vi "Configure Channel Binding.vi"(8 "error in (no error)":errorcluster, 9 "NIVS.System Definition Root":refnum<k24>, 11 "Data cluster in":T1) -> (0 "error out":errorcluster, 3 "Data cluster out":T1)   [LabVIEW 2013]
doc: "Use this template to create a dialog box with event handling."
uses:
  <vilib>/NI Veristand/UI Controls/Single Node Browser/NI_VS UI Single Node Browser.lvlib
  NationalInstruments.VeriStand.SystemStorage
  Support/PWM Object Parameters.ctl
  NationalInstruments.VeriStand.SystemStorageUI
panel:
  in  "RIO?":bool caption="Hardware type - click to toggle"
  in  "Cancel":bool
  in  "Ok":bool
  in  "Selected Channel":refnum<k24>(container)
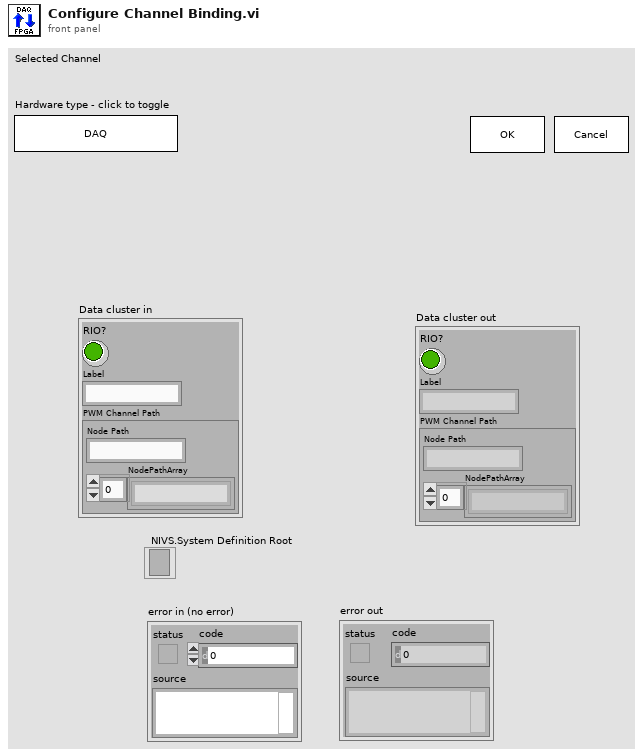
[diagram p1: front panel]
types:
  T1 = typedef "PWM Object Parameters.ctl" = cluster{"RIO?":bool, "Label":string, "PWM Channel Path":cluster{"NodePathArray":string[], "Node Path":string}}
  T2 = typedef "NI_VS UI Single Node Browser.lvlib/Callback Type.ctl" = cluster{"Net Callbacks":refnum<k27>[], "Event":refnum<user-event>}
  T3 = typedef "NI_VS UI Single Node Browser.lvlib/Node Ref.ctl" = refnum<k24>
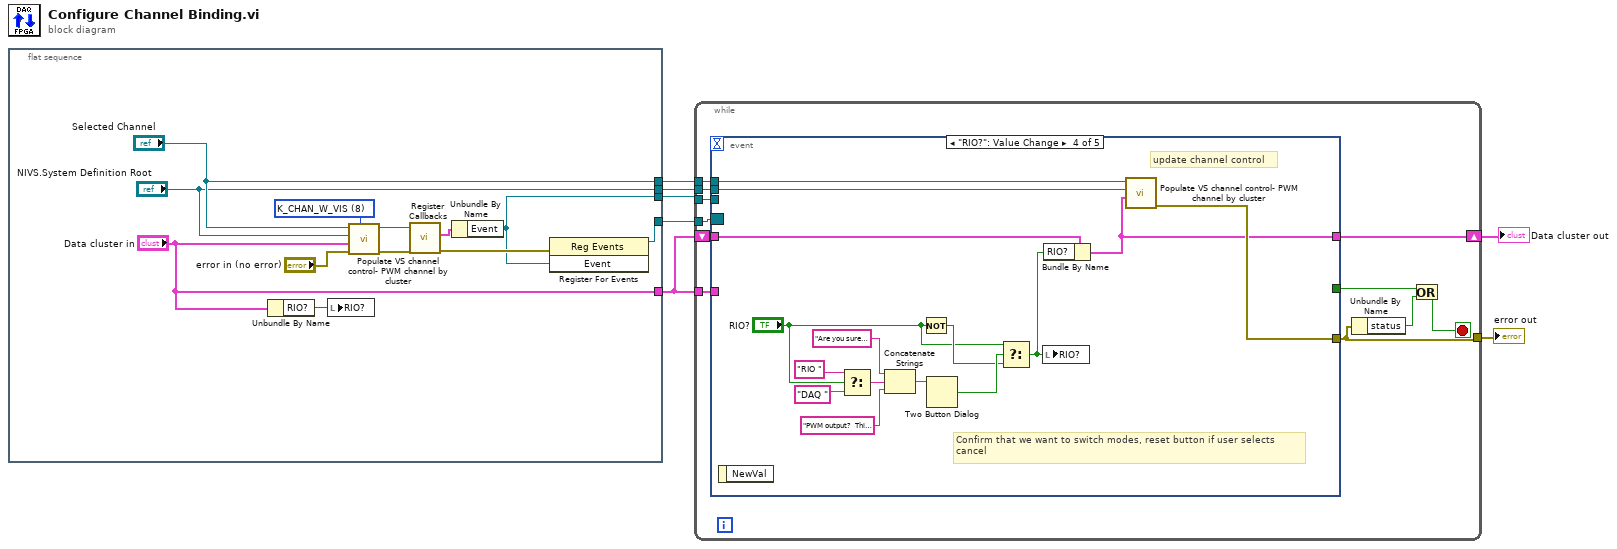
[diagram p0: block diagram]
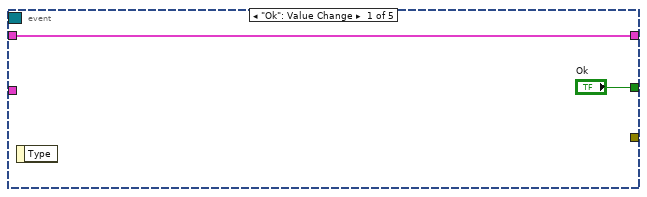
[diagram p2: hidden frame]
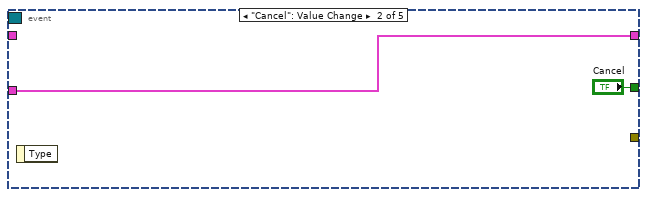
[diagram p3: hidden frame]
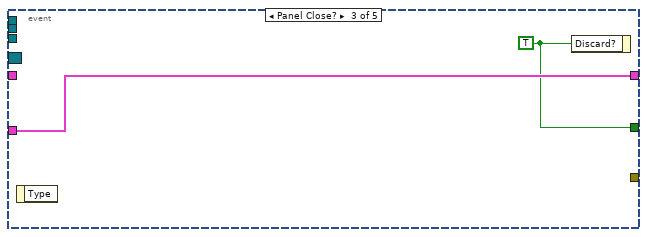
[diagram p4: hidden frame]
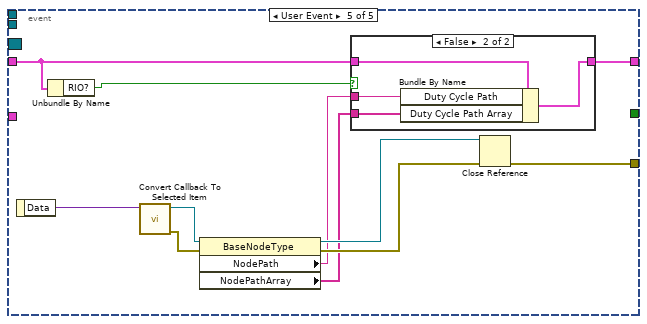
[diagram p5: hidden frame]
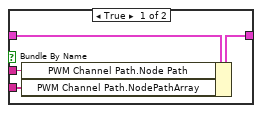
[diagram p6: hidden frame]
diagram:
  n1 = flat-sequence {
    tunnel: [w18] -> w6
    tunnel: [w13] -> w4
    tunnel: ["Selected Channel"] -> w3
    tunnel: ["NIVS.System Definition Root"] -> w2
    tunnel: ["Data cluster in"] -> w1
    frame #0 {
      w10 = u8 8 items=["K_CHAN_R", "K_CHAN_W", "K_CHAN_RW", "K_CHAN_VOLT", "K_CHAN_FAULT", "K_ALL", "K_CUSTOM", "K_CHAN_R_VIS", "K_CHAN_W_VIS", "K_CHAN_RW_VIS", "K_CHAN_VOLT_VIS", "K_CHAN_FAULT_VIS"] ("DisplayFilter")
      n2 = Unbundle By Name("Data cluster in") -> ("RIO?"=w8:bool)
      n3 = local write "RIO?"(w8) -> ()
      n4 = call "Populate VS channel control- PWM channel by cluster.vi"("DisplayFilter"=w10, "error in (no error)"="error in (no error)", "Data cluster in"="Data cluster in", "NIVS.System Definition Root"="NIVS.System Definition Root", ".NET Refnum in"="Selected Channel") -> ("error out"=w15:errorcluster, ".NET Refnum out"=w14:refnum<k24>)  [unwired: 5 in]
      n5 = call <vilib>:"Register Callbacks.vi"("error in (no error)"=w15, "Single Node Browser"=w14) -> ("error out"=w19:errorcluster, "Callbacks"=w16:T2)  [unwired: 7 in, 1 out]
      n6 = Unbundle By Name(w16) -> ("Event"=w13:refnum<user-event>)
      n7 = register-events(error in=w19, w13) -> (reference out=w18:refnum<event-registration>)  [unwired: 1 in, 1 out]
    }
  }
  n8 = while {
    tunnel: [w29] -> w7
    tunnel: w6 -> [w27]
    shift-right: [w24] -> w5
    shift-left: w1 -> [w26]
    tunnel: w1 -> [w25]
    tunnel: w4 -> [w22]
    tunnel: w3 -> [w21]
    tunnel: w2 -> [w20]
    stop <- w23 stop-if-true
    n9 = event shown="[3] \"RIO?\": Value Change" {
      selector: w27 -> [_ _ _ _ _]
      dyn-events: _ -> [_ _ _ _ _]
      timeout: _ -> [_ _ _ _ _]
      tunnel: ["Ok" "Cancel" w35 _ _] -> w30
      tunnel: [_ _ _ w44 w61] -> w29
      tunnel: w26 -> [w31 _ _ w45 w53]
      tunnel: w25 -> [_ w33 w36 _ _]
      tunnel: [w31 w33 w36 w43 w56] -> w24
      tunnel: w22 -> [_ _ _ _ _]
      tunnel: w21 -> [_ _ _ w47 _]
      tunnel: w20 -> [_ _ _ w46 _]
      event "Ok": Value Change {
        n10 = event-data() -> ()  [unwired: 1 in, 1 out]
      }
      event "Cancel": Value Change {
        n11 = event-data() -> ()  [unwired: 1 in, 1 out]
      }
      event Panel Close? {
        w35 = TRUE ("Cancel")
        n12 = event-data() -> ()  [unwired: 1 in, 1 out]
        n13 = event-data("Discard?"=w35) -> ()  [unwired: 1 in, 1 out]
      }
      event "RIO?": Value Change {
        # "update channel control"
        # "Confirm that we want to switch modes, reset button if user selects\ncancel"
        n14 = event-data() -> ()  [unwired: 1 in, 1 out]
        n15 = Select(t="RIO ", s="RIO?", f="DAQ ") -> (s? t:f=w40:string)
        n16 = Concatenate Strings("Are you sure you want to change this channel binding to " ("string"), w40, "PWM output?  This will change the required duty cycle format." ("string")) -> (w49:string)
        n17 = Not(x="RIO?") -> (.not. x?=w38:bool)
        n18 = Two Button Dialog(message=w49) -> (T button?=w48:bool)  [unwired: 2 in]
        n19 = Select(t="RIO?", s=w48, f=w38) -> (s? t:f=w39:bool)
        n20 = local write "RIO?"(w39) -> ()
        n21 = Bundle By Name(cluster=w45, "RIO?"=w39) -> (w43:T1)
        n22 = call "Populate VS channel control- PWM channel by cluster.vi"("Data cluster in"=w43, "NIVS.System Definition Root"=w46, ".NET Refnum in"=w47) -> ("error out"=w44:errorcluster)  [unwired: 7 in, 1 out]
      }
      event User Event {
        n23 = event-data() -> ("Data"=w62:variant)  [unwired: 1 in]
        n24 = Unbundle By Name(w53) -> ("RIO?"=w52:bool)
        n25 = call <vilib>:"Convert Callback To Selected Item.vi"("Data"=w62) -> ("error out"=w57:errorcluster, "Selected Item"=w60:T3)  [unwired: 9 in]
        n26 = property class="BaseNodeType"(reference=w60, error in=w57) -> (reference out=w59:T3, error out=w58:errorcluster, "NodePath"=w55:string, "NodePathArray"=w54:string[])
        n27 = case shown="False" w52 {
          tunnel: [w66 w70] -> w56
          tunnel: w53 -> [w65 w69]
          tunnel: w55 -> [w64 w68]
          tunnel: w54 -> [w63 w67]
          frame True {
            n28 = Bundle By Name(cluster=w65, "PWM Channel Path.Node Path"=w64, "PWM Channel Path.NodePathArray"=w63) -> (w66:T1)
          }
          frame False {
            n29 = Bundle By Name(cluster=w69, "Duty Cycle Path"=w68, "Duty Cycle Path Array"=w67) -> (w70:T1)
          }
        }
        n30 = Close Reference(reference=w59, error in (no error)=w58) -> (error out=w61:errorcluster)
      }
    }
    n31 = Unbundle By Name(w29) -> ("status"=w28:bool)
    n32 = Or(x=w30, y=w28) -> (x .or. y?=w23:bool)
  }
  "error out" <- w7
  "Data cluster out" <- w5
